vi "Display and Log Count Traces.vi"(5 "Record stab":bool, 7 "Laser power in":dbl, 11 "TraceData in":dbl[][](array[numeric]), 13 "Integration time (ms)":T1, 17 "PDM2 ctr in":dbl, 18 "PDM1 ctr in":dbl, 19 "SPCM ctr in":dbl) -> (0 "PDM2 counts":i32=700, 2 "PDM1 trace":dbl(graph)=40.0, 6 "PDM2 trace":dbl(graph), 8 "Trace Data out":dbl[][](array[numeric]), 10 "All Detector Counts":dbl[][](graph)=[[0.0, 220400.0, 219240.0, 225830.0, 224890.0, 223810.0, 225460.0, 238050.0, 225110.0, 232890.0, 227050.0, 222660.0, 239150.0, 227940.0, 224430.0, 259470.0, 252620.0, 229230.0, 241420.0, 225990.0, 227130.0, 226070.0, 228590.0, 240960.0, 238450.0, 251370.0, 236000.0, 232920.0, 220170.0, 223360.0, 221670.0, 230910.0, 233340.0, 232890.0, 229450.0, 240640.0, 229870.0, 228150.0, 228370.0, 224520.0, 236950.0, 242550.0, 247410.0, 236600.0, 239950.0, 243860.0, 230950.0, 225270.0, 225200.0, 240920.0, 242040.0, 237840.0, 224190.0, 260250.0, 236350.0, 226930.0, 222880.0, 229600.0, 240430.0, 230070.0, 242190.0, 233470.0, 222240.0, 274760.0, 230750.0, 224900.0, 225220.0, 222130.0, 226570.0, 234800.0, 238210.0, 227170.0, 236300.0, 222820.0, 219990.0, 225210.0, 227990.0, 246480.0, 234860.0, 234750.0, 245210.0, 231130.0, 222460.0, 224090.0, 227540.0, 244750.0, 247130.0, 241450.0, 247760.0, 232710.0, 238780.0, 235580.0, 236240.0, 232660.0, 226990.0, 241510.0, 239210.0, 225950.0, 233120.0, 231710.0, 224670.0, 233470.0, 243310.0, 230350.0, 238920.0, 225370.0, 234860.0, 233520.0, 224140.0, 223810.0, 223710.0, 241280.0, 239200.0, 243720.0, 236970.0, 226420.0, 224480.0, 226730.0, 233630.0, 227380.0, 269960.0, 245760.0, 251880.0, 235070.0, 245710.0, 236220.0, 227260.0, 231090.0, 225530.0, 223600.0, 225570.0, 224200.0, 240670.0, 240460.0, 229870.0, 226430.0, 226110.0, 222420.0, 241040.0, 233780.0, 245190.0, 234210.0, 225010.0, 223920.0, 229950.0, 228650.0, 230100.0, 228480.0, 229830.0, 222940.0, 222000.0, 220960.0, 227910.0, 220080.0, 226820.0, 228840.0, 234270.0, 228520.0, 233650.0, 230420.0, 231280.0, 230080.0, 226630.0, 225600.0, 228700.0, 225130.0, 227650.0, 225440.0, 234260.0, 234010.0, 229620.0, 225780.0, 229310.0, 230270.0, 231090.0, 220630.0, 245200.0, 235460.0, 224700.0, 238100.0, 241650.0, 226500.0, 226630.0, 239390.0, 237310.0, 242340.0, 233260.0, 268480.0, 224560.0, 223150.0, 221800.0, 221110.0, 228310.0, 222860.0, 232560.0, 222600.0, 227850.0, 227500.0, 228150.0, 228840.0, 224810.0, 226430.0, 225310.0, 225270.0, 223690.0, 219840.0, 226850.0, 222030.0, 221740.0, 228210.0, 224450.0, 224050.0, 220010.0, 226380.0, 228180.0, 221060.0, 242070.0, 225420.0, 231760.0, 227980.0, 232360.0, 240320.0, 246810.0, 230010.0, 219510.0, 255170.0, 218710.0, 217130.0, 219910.0, 225930.0, 233860.0, 239330.0, 229170.0, 238460.0, 227730.0, 223880.0, 225050.0, 225050.0, 222160.0, 222120.0, 238710.0, 231180.0, 216960.0, 218720.0, 223750.0, 218640.0, 215520.0, 218460.0, 217960.0, 224320.0, 220910.0, 227020.0, 222560.0, 222260.0, 216340.0, 221200.0, 218920.0, 226760.0, 217910.0, 218220.0, 222870.0, 222670.0, 217950.0, 223310.0, 226000.0, 223090.0, 224050.0, 218570.0, 232280.0, 215980.0, 238060.0, 220790.0, 217290.0, 219920.0, 230130.0, 233790.0, 236070.0, 215500.0, 229400.0, 230860.0, 223350.0, 218230.0, 217230.0, 220950.0, 232570.0, 227790.0, 240150.0, 228140.0, 237940.0, 220820.0, 218600.0, 218990.0, 229770.0, 239090.0, 224890.0, 239660.0, 258400.0, 241490.0, 218590.0, 216660.0, 223230.0, 240580.0, 239680.0, 223300.0, 227690.0, 233320.0, 236750.0, 220490.0, 225600.0, 231970.0, 231680.0, 222640.0, 233740.0, 218760.0, 218400.0, 219640.0, 234980.0, 227760.0, 219550.0, 223800.0, 220230.0, 223840.0, 222730.0, 221860.0, 228840.0, 221200.0, 225250.0, 226180.0, 230840.0, 229710.0, 225310.0, 220740.0, 229880.0, 227110.0, 223230.0, 229500.0, 224160.0, 223170.0, 223350.0, 223590.0, 228190.0, 236430.0, 217030.0, 223240.0, 216780.0, 225230.0, 236870.0, 230420.0, 219790.0, 234050.0, 218930.0, 223870.0, 224360.0, 221760.0, 231530.0, 238330.0, 240150.0, 240420.0, 230590.0, 228160.0, 227220.0, 238730.0, 224810.0, 244680.0, 264540.0, 251460.0, 231990.0, 247110.0, 240500.0, 249570.0, 222990.0, 222850.0, 235740.0, 232310.0, 233870.0, 242430.0, 237350.0, 238220.0, 244400.0, 223730.0, 224350.0, 224120.0, 234830.0, 225390.0, 223010.0, 232700.0, 227480.0, 234880.0, 226790.0, 235940.0, 260000.0, 230560.0, 230150.0, 233990.0, 230240.0, 230340.0, 230000.0, 239100.0, 229590.0, 223820.0, 226590.0, 222950.0, 228560.0, 222310.0, 226900.0, 224300.0, 229660.0, 223920.0, 220620.0, 222970.0, 223380.0, 224460.0, 229230.0, 223760.0, 230410.0, 219430.0, 220650.0, 226180.0, 220510.0, 225030.0, 226670.0, 235260.0, 229050.0, 229320.0, 228110.0, 232290.0, 231690.0, 223890.0, 224750.0, 228630.0, 226110.0, 225090.0, 222580.0, 223340.0, 230260.0, 223200.0, 226030.0, 221350.0, 223210.0, 227600.0, 215550.0, 219270.0, 227280.0, 223330.0, 221360.0, 221240.0, 223620.0, 226490.0, 224910.0, 222700.0, 231490.0, 223150.0, 225590.0, 217250.0, 236840.0, 219590.0, 255410.0, 241340.0, 251810.0, 225770.0, 225050.0, 222850.0, 235390.0, 233870.0, 244170.0, 223430.0, 215610.0, 221980.0, 223430.0, 220640.0, 224850.0, 224170.0, 219600.0, 222100.0, 217620.0, 218890.0, 226530.0, 222170.0, 223170.0, 223970.0, 223160.0, 227660.0, 225440.0, 224840.0, 227110.0, 222880.0, 223110.0, 218240.0, 218900.0, 223510.0, 222970.0, 220860.0, 250510.0, 222530.0, 224620.0, 227720.0, 222830.0, 223000.0, 224670.0, 225470.0, 221920.0, 222630.0, 222990.0, 219690.0, 220180.0, 223000.0, 232380.0, 224210.0, 225110.0, 228650.0, 226680.0, 228070.0, 225420.0, 229490.0, 225710.0, 223710.0, 223430.0, 218600.0, 224660.0, 232640.0, 223780.0, 235150.0, 224260.0, 232030.0, 237750.0, 235870.0, 235450.0, 234710.0, 232730.0, 234370.0, 242770.0, 232430.0, 222820.0, 221750.0, 219510.0, 232800.0, 239180.0, 221360.0, 266830.0, 240070.0, 231860.0, 217950.0, 226760.0, 222100.0, 222470.0, 242350.0, 238180.0, 239380.0, 244310.0, 245080.0, 228800.0, 221780.0, 219970.0, 232500.0, 239010.0, 233250.0, 235280.0, 242450.0, 230290.0, 226400.0, 220430.0, 225010.0, 238870.0, 241020.0, 232810.0, 224170.0, 216420.0, 242790.0, 226450.0, 219440.0, 225010.0, 233760.0, 232100.0, 235450.0, 236310.0, 236960.0, 243650.0, 228140.0, 227480.0, 232970.0, 228680.0, 225800.0, 232120.0, 226170.0, 262190.0, 241230.0, 222120.0, 227480.0, 221490.0, 218950.0, 239050.0, 236500.0, 235360.0, 241940.0, 223880.0, 223840.0, 225580.0, 238580.0, 242970.0, 222020.0, 229140.0, 257260.0, 246230.0, 248720.0, 226900.0, 226160.0, 225300.0, 228180.0, 239680.0, 234390.0, 234380.0, 223600.0, 240040.0, 228390.0, 229550.0, 223420.0, 236390.0, 223270.0, 261810.0, 237030.0, 228420.0, 249630.0, 223420.0, 217380.0, 223920.0, 218760.0, 215180.0, 217930.0, 231550.0, 219020.0, 220180.0, 223230.0, 232920.0, 233040.0, 218180.0, 224190.0, 220240.0, 216110.0, 219200.0, 216840.0, 215040.0, 221940.0, 222000.0, 225240.0, 227350.0, 222100.0, 227160.0, 220420.0, 221620.0, 219630.0, 217370.0, 224820.0, 222550.0, 220270.0, 222490.0, 216690.0, 221840.0, 237000.0, 217180.0, 216100.0, 214570.0, 223250.0, 236870.0, 229890.0, 237260.0, 233380.0, 230540.0, 217700.0, 218380.0, 225350.0, 232300.0, 239000.0, 232120.0, 231120.0, 219800.0, 232820.0, 227000.0, 225820.0, 225430.0, 223960.0, 222100.0, 219000.0, 218200.0, 216240.0, 216420.0, 215430.0, 216990.0, 222110.0, 219720.0, 225260.0, 219610.0, 222510.0, 219550.0, 222350.0, 220320.0, 222810.0, 219240.0, 226630.0, 224160.0, 219930.0, 218000.0, 225410.0, 226680.0, 218130.0, 223420.0, 225170.0, 221300.0, 232960.0, 243160.0, 241090.0, 224060.0, 217820.0, 216730.0, 226770.0, 220520.0, 225810.0, 234630.0, 231120.0, 236730.0, 229940.0, 240390.0, 213410.0, 216470.0, 216810.0, 217760.0, 225420.0, 220570.0, 219980.0, 222840.0, 214580.0, 220710.0, 215650.0, 223530.0, 215490.0, 218370.0, 221690.0, 211700.0, 221570.0, 211730.0, 219340.0, 207300.0, 216300.0, 213170.0, 215910.0, 214690.0, 219940.0, 217340.0, 209510.0, 207030.0, 211190.0, 210850.0, 214960.0, 210130.0, 211480.0, 210070.0, 213590.0, 212310.0, 217060.0, 211380.0, 216690.0, 227270.0, 225580.0, 229710.0, 228020.0, 230930.0, 220580.0, 216520.0, 210400.0, 212380.0, 213930.0, 221370.0, 225760.0, 207800.0, 220300.0, 212850.0, 211090.0, 222660.0, 210160.0, 222410.0, 224780.0, 242360.0, 220440.0, 224710.0, 214050.0, 215600.0, 210880.0, 212620.0, 215040.0, 228160.0, 229760.0, 216960.0, 222140.0, 220640.0, 220050.0, 210500.0, 214470.0, 223890.0, 225660.0, 224200.0, 224910.0, 227910.0, 227390.0, 209520.0, 210760.0, 213660.0, 219090.0, 207360.0, 222420.0, 220790.0, 211960.0, 213500.0, 220300.0, 220340.0, 232450.0, 242910.0, 234010.0, 227420.0, 228990.0, 227290.0, 212210.0, 220260.0, 218140.0, 211550.0, 217490.0, 229840.0, 225650.0, 211430.0, 252150.0, 223040.0, 210190.0, 210550.0, 208430.0, 216910.0, 222650.0, 213570.0, 228790.0, 213070.0, 211930.0, 212700.0, 207770.0, 226840.0, 219390.0, 213290.0, 212220.0, 211310.0, 213710.0, 211360.0, 212740.0, 210680.0, 217740.0, 210750.0, 212330.0, 215120.0, 217840.0, 217000.0, 220580.0, 225220.0, 210770.0, 215280.0, 209880.0, 214400.0, 210430.0, 211580.0, 212780.0, 226620.0, 218590.0, 208250.0, 214300.0, 222480.0, 224770.0, 224510.0, 236590.0, 225770.0, 231680.0, 214100.0, 217210.0, 221850.0, 218380.0, 223180.0, 232290.0, 228720.0, 227800.0, 234180.0, 213820.0, 218340.0, 217920.0, 213830.0, 227280.0, 224710.0, 223960.0, 231380.0, 236480.0, 220610.0, 215150.0, 214940.0, 218700.0, 234970.0, 232550.0, 225020.0, 235450.0, 228520.0, 213780.0, 213690.0, 211060.0, 220570.0, 230320.0, 227430.0, 234460.0, 227840.0, 222600.0, 217130.0, 214350.0, 214880.0, 217020.0, 219690.0, 224570.0, 226520.0, 226240.0, 227360.0, 212650.0, 216800.0, 209840.0, 225940.0, 233910.0, 227690.0, 226930.0, 230340.0, 223210.0, 213980.0, 212520.0, 215280.0, 224860.0, 226070.0, 224660.0, 206260.0, 248590.0, 232330.0, 211780.0, 211520.0, 215550.0, 215310.0, 211090.0, 225530.0, 237360.0, 212410.0, 209890.0, 211280.0, 213910.0, 217710.0, 224870.0, 213580.0, 217370.0, 260220.0, 230250.0, 219230.0, 217080.0, 213050.0, 213410.0, 210010.0, 220230.0, 215520.0, 229600.0, 216110.0, 210900.0, 211310.0, 206870.0, 244200.0, 227730.0, 206510.0, 208630.0, 246790.0, 220720.0, 224150.0, 210970.0, 216350.0, 220480.0, 214420.0, 226300.0, 210950.0, 215620.0, 216550.0, 210720.0, 216600.0, 212590.0, 246060.0, 226780.0, 222850.0, 215720.0, 219330.0, 214390.0, 226080.0, 214040.0, 213900.0, 208000.0, 219760.0, 219390.0, 214410.0, 237220.0, 208580.0, 219950.0, 207590.0, 214210.0, 231370.0, 212920.0, 224110.0, 210070.0, 220620.0, 212150.0, 210400.0, 206270.0, 207950.0, 249010.0, 218360.0, 209010.0, 239790.0, 222640.0, 217470.0, 209530.0, 214880.0, 213440.0, 216890.0, 217710.0, 225720.0, 224030.0, 234970.0, 231900.0, 228020.0, 214020.0, 215530.0, 213020.0, 215810.0, 223430.0, 217380.0, 212580.0, 221280.0, 208550.0, 204030.0, 224280.0, 230060.0, 219930.0, 223060.0, 220230.0, 230310.0, 225490.0, 212450.0, 208110.0, 212630.0, 209740.0, 226430.0, 214030.0, 221250.0, 207460.0, 216950.0, 221210.0, 209420.0, 213790.0, 208280.0, 217550.0, 223460.0, 211970.0, 235370.0, 206240.0, 217540.0, 208460.0, 208420.0, 219660.0, 218350.0, 225620.0, 215180.0, 226750.0, 208080.0, 216270.0, 206540.0, 203460.0, 214960.0, 224230.0, 221350.0, 214220.0, 229440.0, 214290.0, 221960.0, 210170.0, 207260.0, 205180.0, 207580.0, 206680.0, 230120.0, 205830.0, 252250.0, 242510.0, 215670.0, 216830.0, 213630.0, 218470.0, 212620.0, 219810.0, 217930.0, 227230.0, 218080.0, 207780.0, 214640.0, 213340.0, 216930.0, 215980.0, 240570.0, 217450.0, 255440.0, 215260.0, 215960.0, 213280.0, 214720.0, 231460.0, 225110.0, 223610.0, 223200.0, 212470.0, 209420.0, 205590.0, 216930.0, 208560.0, 215480.0, 217680.0, 211380.0, 241910.0, 220320.0, 223600.0, 208530.0, 210690.0, 214570.0, 220190.0, 223700.0, 225080.0, 211970.0, 208830.0, 211440.0, 212440.0, 217770.0, 228530.0, 226420.0, 222490.0, 228360.0, 224340.0, 228250.0, 219710.0, 206100.0, 214870.0, 208010.0, 219210.0, 222240.0, 208150.0, 207730.0, 205820.0, 207440.0, 211090.0, 211780.0, 209790.0, 206800.0, 207650.0, 207830.0, 207640.0, 207210.0, 208690.0, 211010.0, 208970.0, 209830.0, 210350.0, 207360.0, 208890.0, 207760.0, 204510.0, 210850.0, 211120.0, 207120.0, 206000.0, 211230.0, 213860.0, 224960.0, 208010.0, 204960.0, 222050.0, 209450.0, 209590.0, 220570.0, 220080.0, 203260.0, 205580.0, 207990.0, 206300.0, 203930.0, 211430.0, 206410.0, 210410.0, 209190.0, 208560.0, 204480.0, 208860.0, 208030.0, 207840.0, 209130.0, 209900.0, 208980.0, 201340.0, 208040.0, 204460.0, 203660.0, 206980.0, 211500.0, 213530.0, 206260.0, 206920.0, 206010.0, 203550.0, 208010.0, 207830.0, 199070.0, 213980.0, 207050.0, 204370.0, 211890.0, 215460.0, 203010.0, 210030.0, 207630.0, 203810.0, 201410.0, 230620.0, 200130.0, 202630.0, 198320.0, 202640.0, 200930.0, 204390.0, 203030.0, 209740.0, 201410.0, 204270.0, 210600.0, 210110.0, 205310.0, 204210.0, 208940.0, 208740.0, 207210.0, 201820.0, 207730.0, 203540.0, 206690.0, 205670.0, 207960.0, 218290.0, 218460.0, 218280.0, 200640.0, 202720.0, 205440.0, 204410.0, 208880.0, 201550.0, 210690.0, 203840.0, 199290.0, 206180.0, 215740.0, 217330.0, 213890.0, 217420.0, 204230.0, 217970.0, 208840.0, 207920.0, 201770.0, 206040.0, 209340.0, 211250.0, 206910.0, 205260.0, 201450.0, 201400.0, 204350.0, 204660.0, 205050.0, 201420.0, 199860.0, 202340.0, 196730.0, 194900.0, 201800.0, 201200.0, 194160.0, 199950.0, 197600.0, 200430.0, 198810.0, 194880.0, 197750.0, 203160.0, 207120.0, 199570.0, 198540.0, 199990.0, 203120.0, 202470.0, 207110.0, 198910.0, 196550.0, 201230.0, 204620.0, 205870.0, 213140.0, 227150.0, 221450.0, 208720.0, 218640.0, 215730.0, 212930.0, 203600.0, 209040.0, 204020.0, 204440.0, 205190.0, 213510.0, 216380.0, 205280.0, 183150.0, 163050.0, 142710.0, 147490.0, 143340.0, 148410.0, 144490.0, 146100.0, 143080.0, 155660.0, 180380.0, 193020.0, 204730.0, 196550.0, 193500.0, 198150.0, 180150.0, 172320.0, 169350.0, 165830.0, 173810.0, 180270.0, 180810.0, 192640.0, 196400.0, 208190.0, 198310.0, 201090.0, 194540.0, 211060.0, 208790.0, 205540.0, 192000.0, 199130.0, 186250.0, 180850.0, 180180.0, 165430.0, 165680.0, 167810.0, 169980.0, 168650.0, 172620.0, 184700.0, 185570.0, 190220.0, 204450.0, 198010.0, 192700.0, 188200.0, 192950.0, 197910.0, 192060.0, 185090.0, 190230.0, 197740.0, 189960.0, 197860.0, 194020.0, 199930.0, 192260.0, 190910.0, 201870.0, 200340.0, 196100.0, 177150.0, 157270.0, 153880.0, 133780.0, 121720.0, 108330.0, 93410.0, 91140.0, 90200.0, 106680.0, 118890.0, 147080.0, 146910.0, 170030.0, 189610.0, 190140.0, 209550.0, 228940.0, 287140.0, 238790.0, 242890.0, 235300.0, 235930.0, 239450.0, 238030.0, 236870.0, 235770.0, 231750.0, 231380.0, 233500.0, 227870.0, 225540.0, 228260.0, 226050.0, 230680.0, 234880.0, 242420.0, 240820.0, 240250.0, 246720.0, 244380.0, 239840.0, 237260.0, 239710.0, 238890.0, 240970.0, 234410.0, 239550.0, 241240.0, 241140.0, 247520.0, 247990.0, 251060.0, 234020.0, 229760.0, 239430.0, 241810.0, 238950.0, 236150.0, 232880.0, 230700.0, 236090.0, 238070.0, 241150.0, 245010.0, 242300.0, 240690.0, 239220.0, 235370.0, 234310.0, 233920.0, 231640.0, 237540.0, 236470.0, 235440.0, 230090.0, 229860.0, 238700.0, 236300.0, 249970.0, 240090.0, 236370.0, 234160.0, 253420.0, 251900.0, 261230.0, 255500.0, 254040.0, 252330.0, 243420.0, 235420.0, 237610.0, 259430.0, 244690.0, 252190.0, 239000.0, 255240.0, 253340.0, 241730.0, 240750.0, 246630.0, 252130.0, 272360.0, 253720.0, 252760.0, 245300.0, 262290.0, 237180.0, 239110.0, 237330.0, 241950.0]], 12 "SPCM trace":dbl(graph)=5950.0, 14 "SPCM counts":i32=5950, 16 "PDM1 counts":i32=40)   [LabVIEW 2023]
uses:
  Control 1.ctl
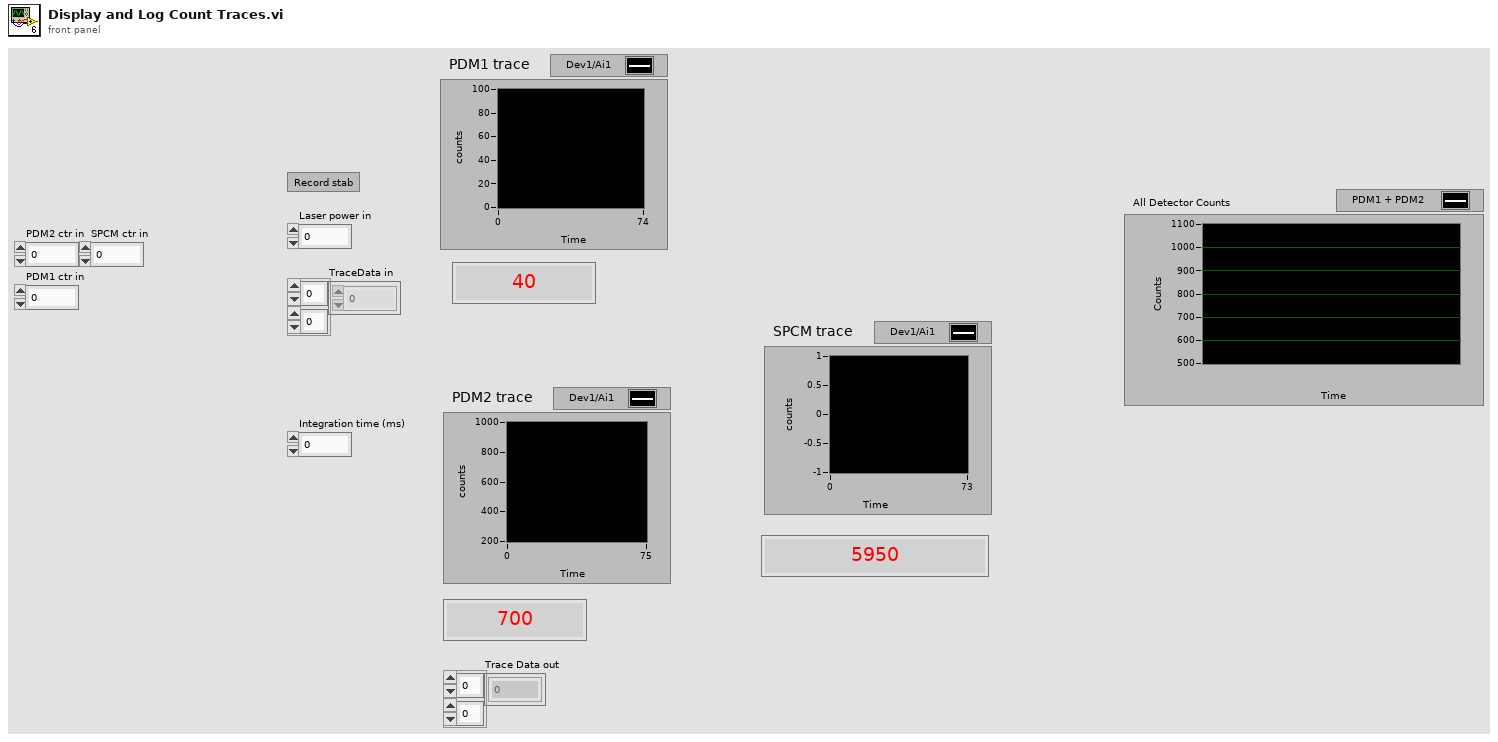
[diagram p1: front panel]
types:
  T1 = typedef "Control 1.ctl" = u32
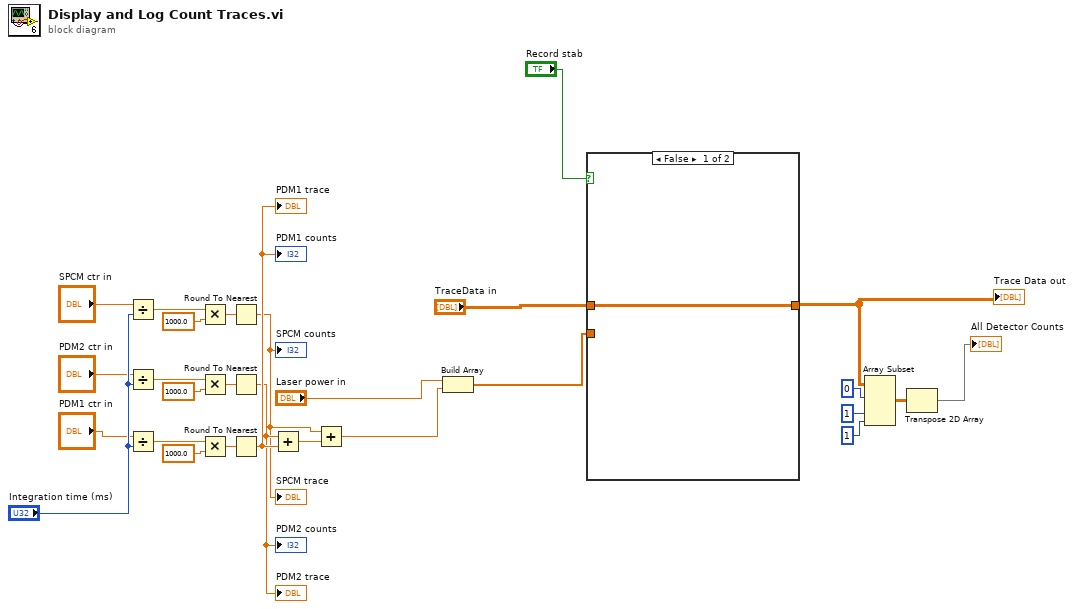
[diagram p0: block diagram]
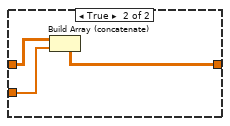
[diagram p2: hidden frame]
diagram:
  n1 = Divide(x="SPCM ctr in", y="Integration time (ms)") -> (x/y=w18:dbl)
  n2 = Divide(x="PDM2 ctr in", y="Integration time (ms)") -> (x/y=w25:dbl)
  n3 = Divide(x="PDM1 ctr in", y="Integration time (ms)") -> (x/y=w20:dbl)
  n4 = Multiply(x=w18, y=1000.0) -> (x*y=w10:dbl)
  n5 = Multiply(x=w25, y=1000.0) -> (x*y=w26:dbl)
  n6 = Multiply(x=w20, y=1000.0) -> (x*y=w11:dbl)
  n7 = Round To Nearest(number=w10) -> (nearest integer value=w8:dbl)
  "SPCM counts" <- w8
  "SPCM trace" <- w8
  n8 = Round To Nearest(number=w26) -> (nearest integer value=w15:dbl)
  "PDM2 counts" <- w15
  "PDM2 trace" <- w15
  n9 = Round To Nearest(number=w11) -> (nearest integer value=w16:dbl)
  "PDM1 counts" <- w16
  "PDM1 trace" <- w16
  n10 = Add(x=w15, y=w16) -> (x+y=w9:dbl)
  n11 = Add(x=w8, y=w9) -> (x+y=w7:dbl)
  n12 = Build Array("Laser power in", w7) -> (w23:dbl[])
  n13 = case shown="False" "Record stab" {
    tunnel: "TraceData in" -> [w29 w32]
    tunnel: w23 -> [_ w31]
    tunnel: [w29 w30] -> w5
    frame False {
    }
    frame True {
      n14 = Build Array (concatenate)(w32, w31) -> (w30:dbl[][])
    }
  }
  "Trace Data out" <- w5
  n15 = Array Subset(array=w5, index (row)=0 ("index"), index (col)=1 ("index"), length (col)=1 ("length")) -> (w6:dbl[][])  [unwired: 1 in]
  n16 = Transpose 2D Array(2D array=w6) -> (transposed array=→"All Detector Counts":dbl[][])
